vi "Write Config.vi"(6 "Stroke Calibration":string, 7 "CALIBRATION PARAMETERS":string[](array[string]), 8 "error in (no error)":errorcluster, 9 "STROKE PARAMETERS":dbl[](array[numeric]), 10 "ADC PARAMETERS":dbl[](array[numeric]), 11 "PID  PARAMETERS":dbl[](array[numeric])) -> (0 "error out":errorcluster)   [LabVIEW 2025]
uses:
  Config file  FGV adv enum.ctl
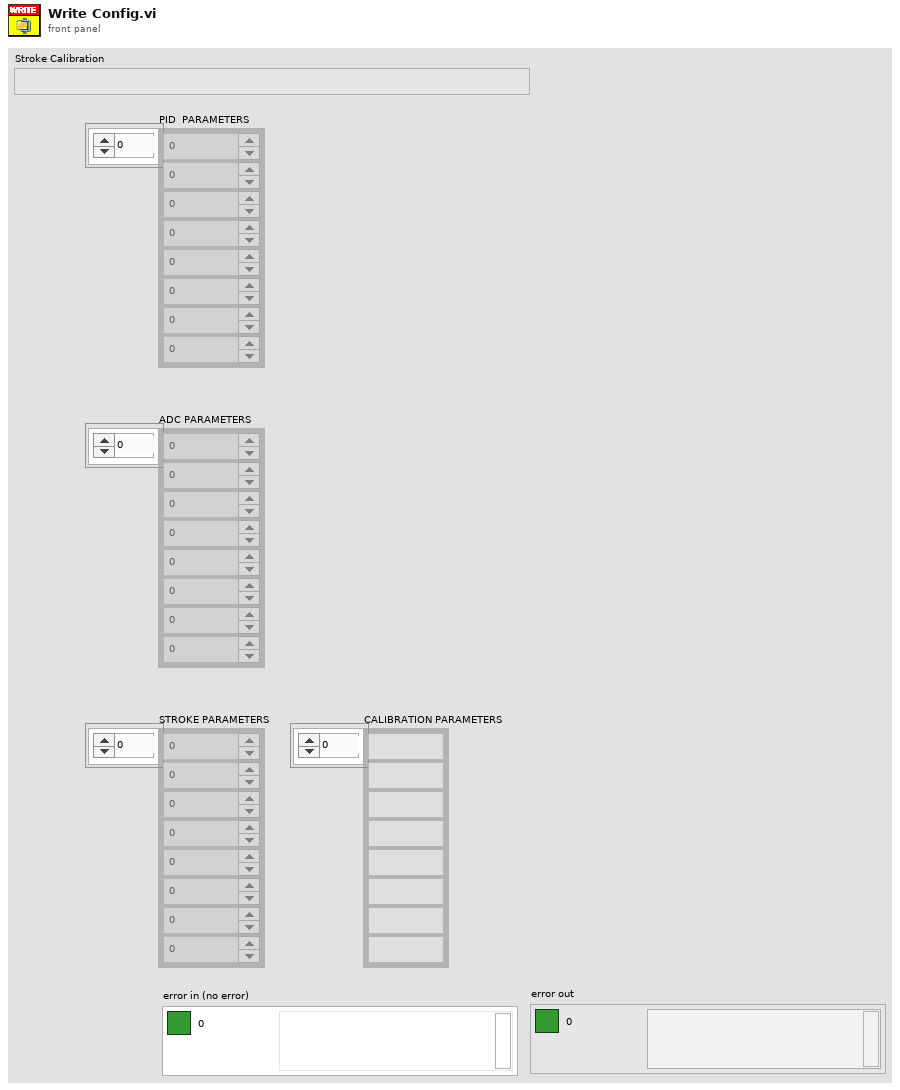
[diagram p1: front panel]
types:
  T1 = typedef "Config file  FGV adv enum.ctl" = enum16{"OPEN", "READ", "WRITE", "CLOSE"}
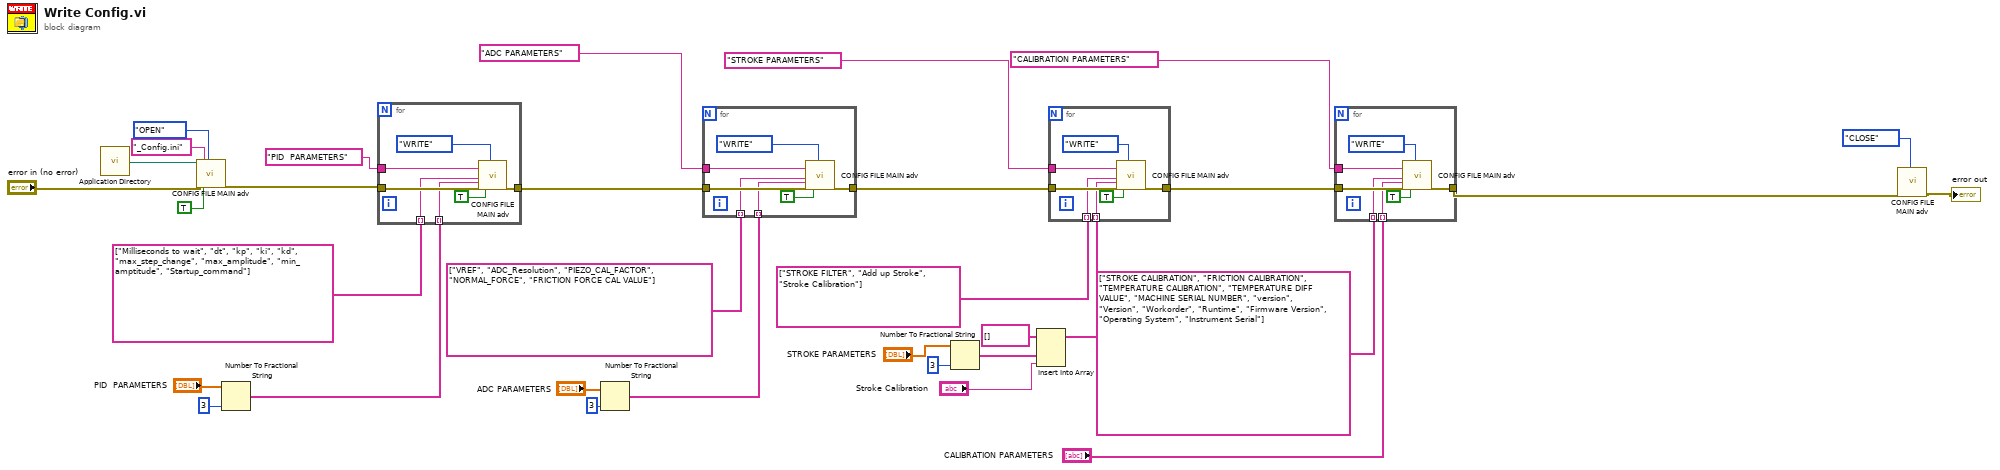
[diagram p0: block diagram]
diagram:
  n1 = call <vilib>:"Application Directory.vi"() -> ("Application Directory"=w27:path)
  n2 = call "CONFIG FILE MAIN adv.vi"("File Path"=w27, "error in"="error in (no error)", "file name"="_Config.ini", "PARAMETER/CONFIG"=TRUE, "Config Enum"=Config_file__FGV_adv_enum."OPEN") -> ("error out"=w26:errorcluster)  [unwired: 13 in, 1 out]
  n3 = Number To Fractional String(number="PID  PARAMETERS", precision (6)=i16 3) -> (F-format string=w16:string[])  [unwired: 2 in]
  n4 = for {
    tunnel: w26 -> [w39]
    tunnel: "PID  PARAMETERS" ("WRITE /READ SECTION") -> [w38]
    tunnel: string[] ["Milliseconds to wait", "dt", "kp", "ki", "kd", "max_step_change", "max_amplitude", "min_amptitude", "Startup_command"] -> [w35] mode=indexing
    tunnel: [w37] -> w23
    tunnel: w16 -> [w34] mode=indexing
    n5 = call "CONFIG FILE MAIN adv.vi"("WRITE /READ SECTION"=w38, "WRITE KEY"=w35, "WRITE VALUE"=w34, "error in"=w39, "PARAMETER/CONFIG"=TRUE, "Config Enum"=Config_file__FGV_adv_enum."WRITE") -> ("error out"=w37:errorcluster)  [unwired: 12 in, 1 out]
  }
  n6 = Number To Fractional String(number="ADC PARAMETERS", precision (6)=i16 3) -> (F-format string=w12:string[])  [unwired: 2 in]
  n7 = for {
    tunnel: w23 -> [w46]
    tunnel: "ADC PARAMETERS" ("WRITE /READ SECTION") -> [w45]
    tunnel: [w44] -> w20
    tunnel: string[] ["VREF", "ADC_Resolution", "PIEZO_CAL_FACTOR", "NORMAL_FORCE", "FRICTION FORCE CAL VALUE"] -> [w42] mode=indexing
    tunnel: w12 -> [w41] mode=indexing
    n8 = call "CONFIG FILE MAIN adv.vi"("WRITE /READ SECTION"=w45, "WRITE KEY"=w42, "WRITE VALUE"=w41, "error in"=w46, "PARAMETER/CONFIG"=TRUE, "Config Enum"=Config_file__FGV_adv_enum."WRITE") -> ("error out"=w44:errorcluster)  [unwired: 12 in, 1 out]
  }
  n9 = Number To Fractional String(number="STROKE PARAMETERS", precision (6)=i16 3) -> (F-format string=w10:string[])  [unwired: 2 in]
  n10 = Insert Into Array(array=string[] [], new element #1=w10, new element #2="Stroke Calibration") -> (w6:string[])  [unwired: 1 in]
  n11 = for {
    tunnel: w20 -> [w53]
    tunnel: "STROKE PARAMETERS" ("WRITE /READ SECTION") -> [w52]
    tunnel: [w51] -> w5
    tunnel: string[] ["STROKE FILTER", "Add up Stroke", "Stroke Calibration"] -> [w49] mode=indexing
    tunnel: w6 -> [w48] mode=indexing
    n12 = call "CONFIG FILE MAIN adv.vi"("WRITE /READ SECTION"=w52, "WRITE KEY"=w49, "WRITE VALUE"=w48, "error in"=w53, "PARAMETER/CONFIG"=TRUE, "Config Enum"=Config_file__FGV_adv_enum."WRITE") -> ("error out"=w51:errorcluster)  [unwired: 12 in, 1 out]
  }
  n13 = for {
    tunnel: w5 -> [w60]
    tunnel: "CALIBRATION PARAMETERS" ("WRITE /READ SECTION") -> [w59]
    tunnel: [w58] -> w4
    tunnel: string[] ["STROKE CALIBRATION", "FRICTION CALIBRATION", "TEMPERATURE CALIBRATION", "TEMPERATURE DIFF VALUE", "MACHINE SERIAL NUMBER", "version", "Version", "Workorder", "Runtime", "Firmware Version", "Operating System", "Instrument Serial"] -> [w56] mode=indexing
    tunnel: "CALIBRATION PARAMETERS" -> [w55] mode=indexing
    n14 = call "CONFIG FILE MAIN adv.vi"("WRITE /READ SECTION"=w59, "WRITE KEY"=w56, "WRITE VALUE"=w55, "error in"=w60, "PARAMETER/CONFIG"=TRUE, "Config Enum"=Config_file__FGV_adv_enum."WRITE") -> ("error out"=w58:errorcluster)  [unwired: 12 in, 1 out]
  }
  n15 = call "CONFIG FILE MAIN adv.vi"("error in"=w4, "Config Enum"=Config_file__FGV_adv_enum."CLOSE") -> ("error out"=→"error out":errorcluster)  [unwired: 16 in, 1 out]
